vi "ConvertHexToDecimal.vi"(11 "Input String":string="\r       0x8000,0x98f8,0xb0fb,0xc71c,0xda82,0xea6d,0xf641,0xfd89,0xffff,0xfd89,0xf641,0xea6d,0xda82,0xc71c,0xb0fb,0x98f8,0x8000,0x6707,0x4f04,0x38e3,0x257d,0x1592,0x9be,0x276,0x0,0x276,0x9be,0x1592,0x257d,0x38e3,0x4f04,0x6707 \n") -> (3 "Output":u16[](array[numeric]))   [LabVIEW 2019]
panel:
  out "Waveform Graph":u16[](graph)
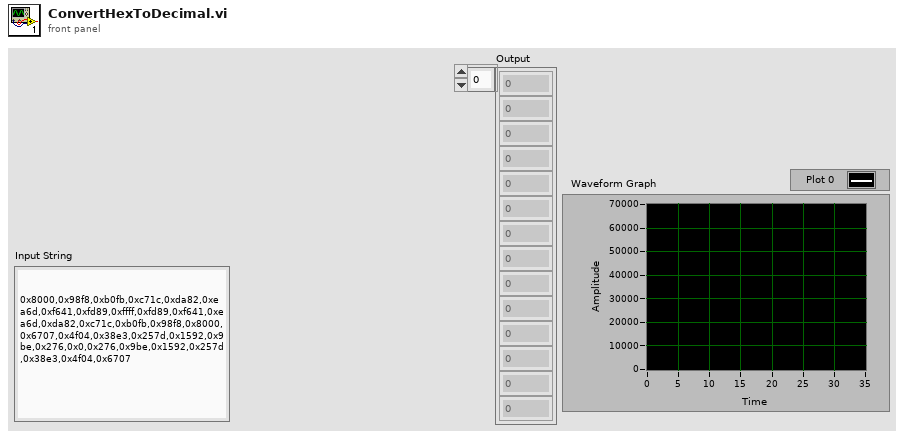
[diagram p1: front panel]
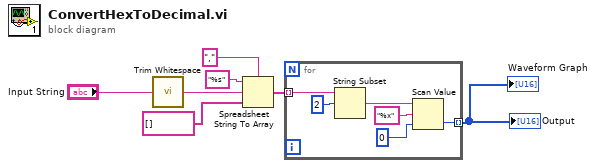
[diagram p0: block diagram]
diagram:
  n1 = call <vilib>:"Trim Whitespace.vi"("string"="Input String") -> ("trimmed string"=w4:string)  [unwired: 1 in]
  n2 = Spreadsheet String To Array(delimiter (Tab)=",", format string="%s", spreadsheet string=w4, array type (2D Dbl)=string[] []) -> (array=w2:string[])
  n3 = for {
    tunnel: w2 -> [w10] mode=indexing
    tunnel: [w11] -> w1 mode=indexing
    n4 = String Subset(string=w10, offset (0)=2) -> (substring=w9:string)  [unwired: 1 in]
    n5 = Scan Value(string=w9, format string="%x", default (0 dbl)=u16 0) -> (value=w11:u16)  [unwired: 1 out]
  }
  "Output" <- w1
  "Waveform Graph" <- w1
